vi "Main GUI.vi"() -> ()   [LabVIEW 2013]
panel:
  in  "Run Experiment":bool
  in  "Experiment Options\nMenu Selector":bool
  in  "Calibration Options\nMenu Selector":bool
  in  "Configuration Options\nMenu Selector":bool
  in  "Experimental Parameters\nMenu Selector":bool
  in  "Persistent Data\nMenu Selector":bool
  in  "Physical Constants\nMenu Selector":bool
  in  "IO Channel \nMenu Selector":bool
  in  "Slope Calibration\nSelector":bool
  in  "Power Peak\nCalibration Selector":bool
  in  "Experiment Execution\nSelector":bool
  in  "Experiment Type\nSelector":bool
  in  "Enforce Set-Points":bool
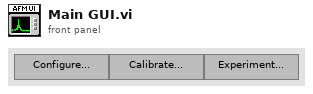
[diagram p1: front panel]
types:
  T1 = cluster{"Set Point Sliders":refnum<vi>, refnum<vi>}
  T2 = cluster{"Sensor State Indicators":refnum<vi>, refnum<vi>}
  T3 = cluster{"IO Channels Menu":refnum<vi>, refnum<vi>}
  T4 = cluster{"Physical Constants Menu":refnum<vi>, refnum<vi>}
  T5 = cluster{"Persistent Data Menu":refnum<vi>, refnum<vi>}
  T6 = cluster{"Experimental Parameters Menu":refnum<vi>, refnum<vi>}
  T7 = cluster{"Power Peak Calibration":refnum<vi>, refnum<vi>}
  T8 = cluster{"Experiment Selector Pane":refnum<vi>, refnum<vi>}
  T9 = cluster{"Deviation Chart":refnum<vi>, refnum<vi>}
  T10 = cluster{"Deviation Chart":refnum<vi>, refnum<vi>}[]
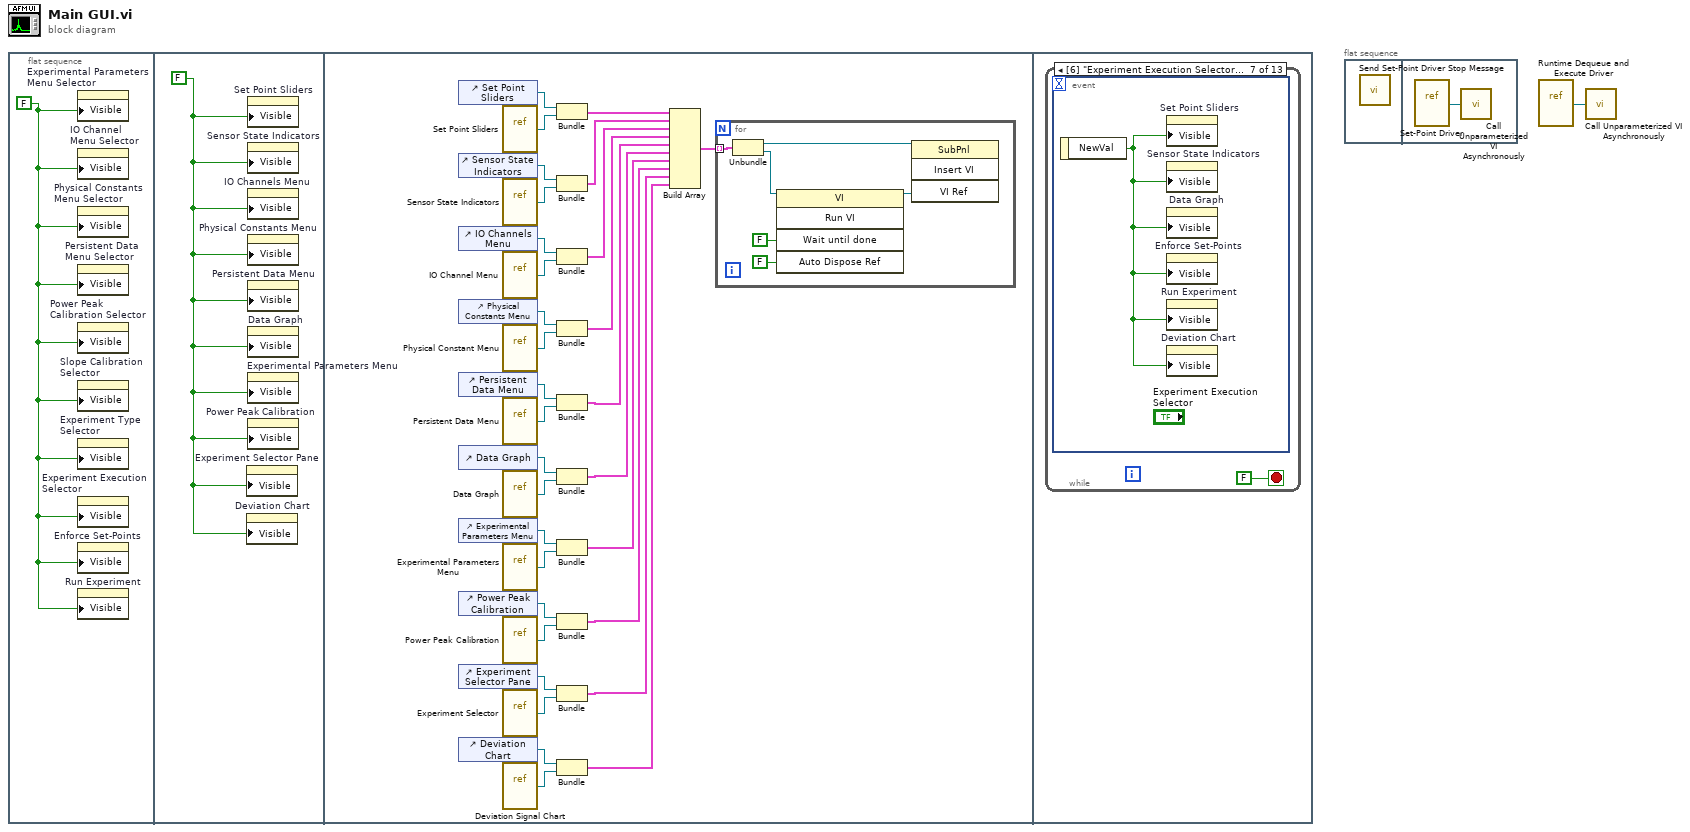
[diagram p0: block diagram]
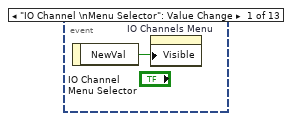
[diagram p2: hidden frame]
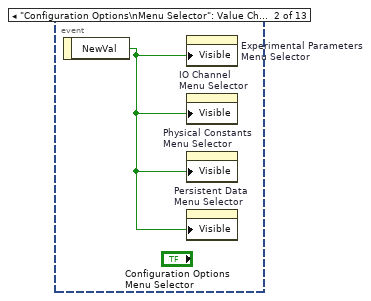
[diagram p3: hidden frame]
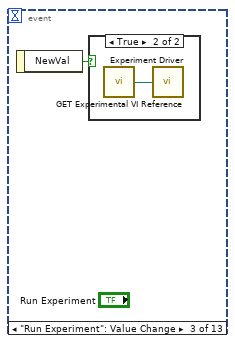
[diagram p4: hidden frame]
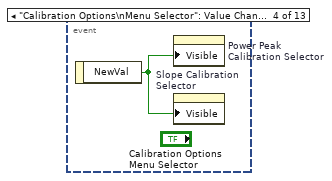
[diagram p6: hidden frame]
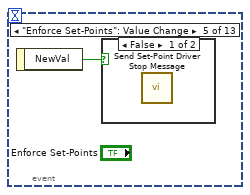
[diagram p7: hidden frame]
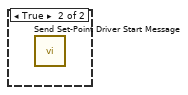
[diagram p8: hidden frame]
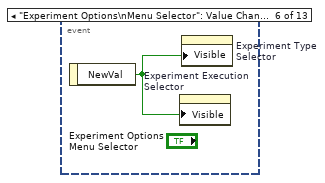
[diagram p9: hidden frame]
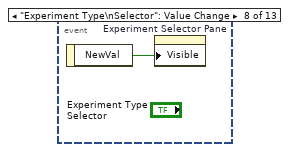
[diagram p10: hidden frame]
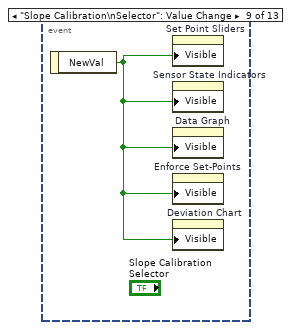
[diagram p11: hidden frame]
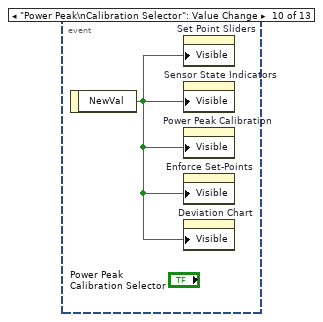
[diagram p12: hidden frame]
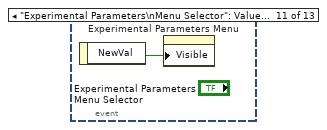
[diagram p13: hidden frame]
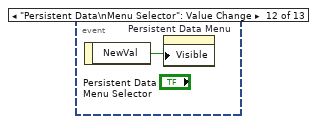
[diagram p14: hidden frame]
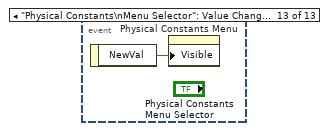
[diagram p15: hidden frame]
diagram:
  n1 = flat-sequence {
    frame #0 {
      w2 = FALSE ("Visible")
      n2 = property on="Experimental Parameters\nMenu Selector" class="Bool (strict)"("Visible"=w2) -> ()  [unwired: 2 in, 2 out]
      n3 = property on="IO Channel \nMenu Selector" class="Bool (strict)"("Visible"=w2) -> ()  [unwired: 2 in, 2 out]
      n4 = property on="Physical Constants\nMenu Selector" class="Bool (strict)"("Visible"=w2) -> ()  [unwired: 2 in, 2 out]
      n5 = property on="Persistent Data \nMenu Selector" class="Bool (strict)"("Visible"=w2) -> ()  [unwired: 2 in, 2 out]
      n6 = property on="Power Peak\nCalibration Selector" class="Bool (strict)"("Visible"=w2) -> ()  [unwired: 2 in, 2 out]
      n7 = property on="Slope Calibration\nSelector" class="Bool (strict)"("Visible"=w2) -> ()  [unwired: 2 in, 2 out]
      n8 = property on="Experiment Type\nSelector" class="Bool (strict)"("Visible"=w2) -> ()  [unwired: 2 in, 2 out]
      n9 = property on="Experiment Execution\nSelector" class="Bool (strict)"("Visible"=w2) -> ()  [unwired: 2 in, 2 out]
      n10 = property on="Enforce Set-Points" class="Bool (strict)"("Visible"=w2) -> ()  [unwired: 2 in, 2 out]
      n11 = property on="Run Experiment" class="Bool"("Visible"=w2) -> ()  [unwired: 2 in, 2 out]
    }
    frame #1 {
      w3 = FALSE ("Visible")
      n12 = property on="Experiment Selector Pane" class="SubPnl"("Visible"=w3) -> ()  [unwired: 2 in, 2 out]
      n13 = property on="Deviation Chart" class="SubPnl"("Visible"=w3) -> ()  [unwired: 2 in, 2 out]
      n14 = property on="Set Point Sliders" class="SubPnl"("Visible"=w3) -> ()  [unwired: 2 in, 2 out]
      n15 = property on="Sensor State Indicators" class="SubPnl"("Visible"=w3) -> ()  [unwired: 2 in, 2 out]
      n16 = property on="IO Channels Menu" class="SubPnl"("Visible"=w3) -> ()  [unwired: 2 in, 2 out]
      n17 = property on="Physical Constants Menu" class="SubPnl"("Visible"=w3) -> ()  [unwired: 2 in, 2 out]
      n18 = property on="Persistent Data Menu" class="SubPnl"("Visible"=w3) -> ()  [unwired: 2 in, 2 out]
      n19 = property on="Data Graph" class="SubPnl"("Visible"=w3) -> ()  [unwired: 2 in, 2 out]
      n20 = property on="Experimental Parameters Menu" class="SubPnl"("Visible"=w3) -> ()  [unwired: 2 in, 2 out]
      n21 = property on="Power Peak Calibration" class="SubPnl"("Visible"=w3) -> ()  [unwired: 2 in, 2 out]
    }
    frame #2 {
      n22 = control-ref of="Set Point Sliders"() -> (w33:refnum<vi>)
      n23 = control-ref of="Sensor State Indicators"() -> (w31:refnum<vi>)
      n24 = control-ref of="IO Channels Menu"() -> (w29:refnum<vi>)
      n25 = control-ref of="Physical Constants Menu"() -> (w27:refnum<vi>)
      n26 = control-ref of="Persistent Data Menu"() -> (w25:refnum<vi>)
      n27 = control-ref of="Data Graph"() -> (w23:refnum<vi>)
      n28 = control-ref of="Experimental Parameters Menu"() -> (w21:refnum<vi>)
      n29 = control-ref of="Power Peak Calibration"() -> (w19:refnum<vi>)
      n30 = control-ref of="Experiment Selector Pane"() -> (w17:refnum<vi>)
      n31 = control-ref of="Deviation Chart"() -> (w5:refnum<vi>)
      n32 = vi-ref "Set Point Sliders.vi"() -> (w32:refnum<vi>)
      n33 = vi-ref "Sensor State Indicators.vi"() -> (w30:refnum<vi>)
      n34 = vi-ref "IO Channel Menu.vi"() -> (w28:refnum<vi>)
      n35 = vi-ref "Physical Constant Menu.vi"() -> (w26:refnum<vi>)
      n36 = vi-ref "Persistent Data Menu.vi"() -> (w24:refnum<vi>)
      n37 = vi-ref "Data Graph.vi"() -> (w22:refnum<vi>)
      n38 = vi-ref "Experimental Parameters Menu.vi"() -> (w20:refnum<vi>)
      n39 = vi-ref "Power Peak Calibration.vi"() -> (w18:refnum<vi>)
      n40 = vi-ref "Experiment Selector.vi"() -> (w16:refnum<vi>)
      n41 = vi-ref "Deviation Signal Chart.vi"() -> (w6:refnum<vi>)
      n42 = Bundle("Set Point Sliders"=w33, w32) -> (w34:T1)  [unwired: 1 in]
      n43 = Bundle("Sensor State Indicators"=w31, w30) -> (w14:T2)  [unwired: 1 in]
      n44 = Bundle("IO Channels Menu"=w29, w28) -> (w13:T3)  [unwired: 1 in]
      n45 = Bundle("Physical Constants Menu"=w27, w26) -> (w12:T4)  [unwired: 1 in]
      n46 = Bundle("Persistent Data Menu"=w25, w24) -> (w11:T5)  [unwired: 1 in]
      n47 = Bundle("Data Graph"=w23, w22) -> (w10:cluster{"Data Graph":refnum<vi>, refnum<vi>})  [unwired: 1 in]
      n48 = Bundle("Experimental Parameters Menu"=w21, w20) -> (w9:T6)  [unwired: 1 in]
      n49 = Bundle("Power Peak Calibration"=w19, w18) -> (w8:T7)  [unwired: 1 in]
      n50 = Bundle("Experiment Selector Pane"=w17, w16) -> (w7:T8)  [unwired: 1 in]
      n51 = Bundle("Deviation Chart"=w5, w6) -> (w4:T9)  [unwired: 1 in]
      n52 = Build Array(w34, w14, w13, w12, w11, w10, w9, w8, w7, w4) -> (w15:T10)
      n53 = for {
        tunnel: w15 -> [w40] mode=indexing
        n54 = Unbundle(w40) -> ("Deviation Chart"=w39:refnum<vi>, w38:refnum<vi>)
        n55 = invoke class="VI" method="Run VI"(reference=w38, "Wait until done"=FALSE ("Wait Until Done"), "Auto Dispose Ref"=FALSE ("Auto Dispose Reference")) -> (reference out=w37:refnum<vi>)  [unwired: 2 in, 4 out]
        n56 = invoke class="SubPnl" method="Insert VI"(reference=w39, "VI Ref"=w37) -> ()  [unwired: 2 in, 4 out]
      }
    }
    frame #3 {
      n57 = while {
        stop <- FALSE stop-if-true
        n58 = event shown="[6] \"Experiment Execution Selector\": Value Change" {
          selector: _ -> [_ _ _ _ _ _ _ _ _ _ _ _ _]
          dyn-events: _ -> [_ _ _ _ _ _ _ _ _ _ _ _ _]
          timeout: _ -> [_ _ _ _ _ _ _ _ _ _ _ _ _]
          event "IO Channel \nMenu Selector": Value Change {
            n59 = event-data() -> ("NewVal"=w42:bool)  [unwired: 1 in]
            n60 = property on="IO Channels Menu" class="SubPnl"("Visible"=w42) -> ()  [unwired: 2 in, 2 out]
          }
          event "Configuration Options\nMenu Selector": Value Change {
            n61 = event-data() -> ("NewVal"=w43:bool)  [unwired: 1 in]
            n62 = property on="Experimental Parameters\nMenu Selector" class="Bool (strict)"("Visible"=w43) -> ()  [unwired: 2 in, 2 out]
            n63 = property on="IO Channel \nMenu Selector" class="Bool (strict)"("Visible"=w43) -> ()  [unwired: 2 in, 2 out]
            n64 = property on="Physical Constants\nMenu Selector" class="Bool (strict)"("Visible"=w43) -> ()  [unwired: 2 in, 2 out]
            n65 = property on="Persistent Data\nMenu Selector" class="Bool (strict)"("Visible"=w43) -> ()  [unwired: 2 in, 2 out]
          }
          event "Run Experiment": Value Change {
            n66 = event-data() -> ("NewVal"=w44:bool)  [unwired: 1 in]
            n67 = case shown="True" w44 {
              frame False {
              }
              frame True {
                n68 = call "GET Experimental VI Reference.vi"() -> ("Experimental VI Reference"=w45:refnum<vi>)
                n69 = call "Experiment Driver.vi"("Experiment VI Reference"=w45) -> ()
              }
            }
          }
          event "Calibration Options\nMenu Selector": Value Change {
            n70 = event-data() -> ("NewVal"=w46:bool)  [unwired: 1 in]
            n71 = property on="Power Peak\nCalibration Selector" class="Bool (strict)"("Visible"=w46) -> ()  [unwired: 2 in, 2 out]
            n72 = property on="Slope Calibration\nSelector" class="Bool (strict)"("Visible"=w46) -> ()  [unwired: 2 in, 2 out]
          }
          event "Enforce Set-Points": Value Change {
            n73 = event-data() -> ("NewVal"=w47:bool)  [unwired: 1 in]
            n74 = case shown="False" w47 {
              frame False {
                n75 = call "Send Set-Point Driver Stop Message.vi"() -> ()  [unwired: 12 in]
              }
              frame True {
                n76 = call "Send Set-Point Driver Start Message.vi"() -> ()  [unwired: 12 in]
              }
            }
          }
          event "Experiment Options\nMenu Selector": Value Change {
            n77 = event-data() -> ("NewVal"=w48:bool)  [unwired: 1 in]
            n78 = property on="Experiment Execution\nSelector" class="Bool (strict)"("Visible"=w48) -> ()  [unwired: 2 in, 2 out]
            n79 = property on="Experiment Type\nSelector" class="Bool (strict)"("Visible"=w48) -> ()  [unwired: 2 in, 2 out]
          }
          event "Experiment Execution\nSelector": Value Change {
            n80 = event-data() -> ("NewVal"=w49:bool)  [unwired: 1 in]
            n81 = property on="Set Point Sliders" class="SubPnl"("Visible"=w49) -> ()  [unwired: 2 in, 2 out]
            n82 = property on="Sensor State Indicators" class="SubPnl"("Visible"=w49) -> ()  [unwired: 2 in, 2 out]
            n83 = property on="Data Graph" class="SubPnl"("Visible"=w49) -> ()  [unwired: 2 in, 2 out]
            n84 = property on="Enforce Set-Points" class="Bool (strict)"("Visible"=w49) -> ()  [unwired: 2 in, 2 out]
            n85 = property on="Run Experiment" class="Bool"("Visible"=w49) -> ()  [unwired: 2 in, 2 out]
            n86 = property on="Deviation Chart" class="SubPnl"("Visible"=w49) -> ()  [unwired: 2 in, 2 out]
          }
          event "Experiment Type\nSelector": Value Change {
            n87 = event-data() -> ("NewVal"=w50:bool)  [unwired: 1 in]
            n88 = property on="Experiment Selector Pane" class="SubPnl"("Visible"=w50) -> ()  [unwired: 2 in, 2 out]
          }
          event "Slope Calibration\nSelector": Value Change {
            n89 = event-data() -> ("NewVal"=w51:bool)  [unwired: 1 in]
            n90 = property on="Set Point Sliders" class="SubPnl"("Visible"=w51) -> ()  [unwired: 2 in, 2 out]
            n91 = property on="Sensor State Indicators" class="SubPnl"("Visible"=w51) -> ()  [unwired: 2 in, 2 out]
            n92 = property on="Data Graph" class="SubPnl"("Visible"=w51) -> ()  [unwired: 2 in, 2 out]
            n93 = property on="Enforce Set-Points" class="Bool (strict)"("Visible"=w51) -> ()  [unwired: 2 in, 2 out]
            n94 = property on="Deviation Chart" class="SubPnl"("Visible"=w51) -> ()  [unwired: 2 in, 2 out]
          }
          event "Power Peak\nCalibration Selector": Value Change {
            n95 = event-data() -> ("NewVal"=w52:bool)  [unwired: 1 in]
            n96 = property on="Set Point Sliders" class="SubPnl"("Visible"=w52) -> ()  [unwired: 2 in, 2 out]
            n97 = property on="Sensor State Indicators" class="SubPnl"("Visible"=w52) -> ()  [unwired: 2 in, 2 out]
            n98 = property on="Power Peak Calibration" class="SubPnl"("Visible"=w52) -> ()  [unwired: 2 in, 2 out]
            n99 = property on="Enforce Set-Points" class="Bool (strict)"("Visible"=w52) -> ()  [unwired: 2 in, 2 out]
            n100 = property on="Deviation Chart" class="SubPnl"("Visible"=w52) -> ()  [unwired: 2 in, 2 out]
          }
          event "Experimental Parameters\nMenu Selector": Value Change {
            n101 = event-data() -> ("NewVal"=w53:bool)  [unwired: 1 in]
            n102 = property on="Experimental Parameters Menu" class="SubPnl"("Visible"=w53) -> ()  [unwired: 2 in, 2 out]
          }
          event "Persistent Data\nMenu Selector": Value Change {
            n103 = event-data() -> ("NewVal"=w54:bool)  [unwired: 1 in]
            n104 = property on="Persistent Data Menu" class="SubPnl"("Visible"=w54) -> ()  [unwired: 2 in, 2 out]
          }
          event "Physical Constants\nMenu Selector": Value Change {
            n105 = event-data() -> ("NewVal"=w55:bool)  [unwired: 1 in]
            n106 = property on="Physical Constants Menu" class="SubPnl"("Visible"=w55) -> ()  [unwired: 2 in, 2 out]
          }
        }
      }
    }
  }
  n107 = flat-sequence {
    frame #0 {
      n108 = call "Send Set-Point Driver Stop Message.vi"() -> ()  [unwired: 12 in]
    }
    frame #1 {
      n109 = vi-ref "Set-Point Driver.vi"() -> (w56:refnum<vi>)
      n110 = call "Call Unparameterized VI Asynchronously.vi"("VI Reference"=w56) -> ()
    }
  }
  n111 = vi-ref "Runtime Dequeue and Execute Driver.vi"() -> (w1:refnum<vi>)
  n112 = call "Call Unparameterized VI Asynchronously.vi"("VI Reference"=w1) -> ()
